vi "插入microwavedata.vi"(7 "pid":i32, 8 "error in":errorcluster, 9 "S-Parameter":dbl[](array[numeric]), 10 "freq":dbl[](array[numeric])) -> (0 "error out":errorcluster)   [LabVIEW 2015]
uses:
  Ctl/DNS.ctl
  Ctl/database_Method.ctl
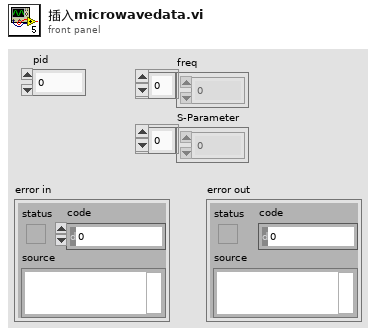
[diagram p1: front panel]
types:
  T1 = typedef "database_Method.ctl" = enum16{"初始化", "查询", "关闭"}
  T2 = typedef "DNS.ctl" = string
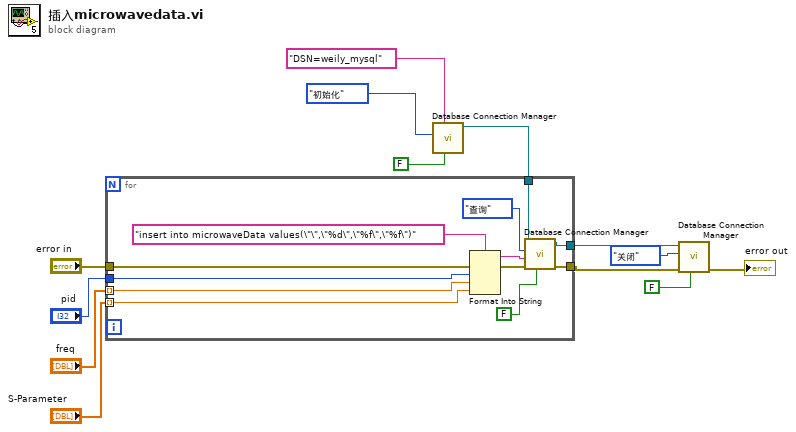
[diagram p0: block diagram]
diagram:
  n1 = call "Database Connection Manager.vi"("Return Data (T)"=FALSE, "ConnectionString"=T2 "DSN=weily_mysql", "Method"=database_Method."初始化") -> ("ADODB._Connection Out"=w6:refnum<k7>)  [unwired: 5 in, 3 out]
  n2 = for {
    tunnel: "freq" -> [w24] mode=indexing
    tunnel: "S-Parameter" -> [w23] mode=indexing
    tunnel: "pid" -> [w22]
    tunnel: [w20] -> w2
    tunnel: "error in" -> [w21]
    tunnel: w6 -> [w15]
    tunnel: [w14] -> w3
    n3 = Format Into String(format string="insert into microwaveData values(\"\",\"%d\",\"%f\",\"%f\")" ("SQL"), error in=w21, w22, w24, w23) -> (resulting string=w18:string, error out=w19:errorcluster)  [unwired: 1 in]
    n4 = call "Database Connection Manager.vi"("Return Data (T)"=FALSE, "error in (no error)"=w19, "Command Text"=w18, "Method"=database_Method."查询", "ADODB._Connection In"=w15) -> ("error out"=w20:errorcluster, "ADODB._Connection Out"=w14:refnum<k7>)  [unwired: 3 in, 2 out]
  }
  n5 = call "Database Connection Manager.vi"("Return Data (T)"=FALSE, "error in (no error)"=w2, "Method"=database_Method."关闭", "ADODB._Connection In"=w3) -> ("error out"=→"error out":errorcluster)  [unwired: 4 in, 3 out]
